vi "LV SciSDK DETACH BOARD.vi"(8 "error in (no error)":errorcluster, 9 "Board Handle In":T1) -> (0 "error out":errorcluster, 1 "SciSDK Handle":u64)   [LabVIEW 2021, in "SciSDK_Labview.lvlib"]
doc: "You need this VI to detach a board from SciSDK"
uses:
  SciSDK_Labview.lvlib
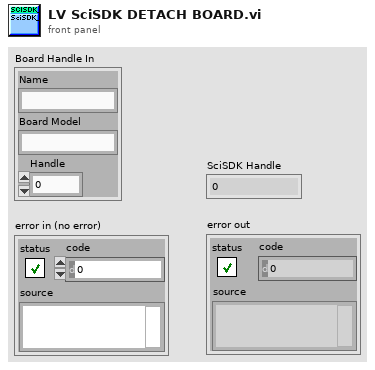
[diagram p1: front panel]
types:
  T1 = cluster{"Name":string, "Board Model":string, "Handle":u64}
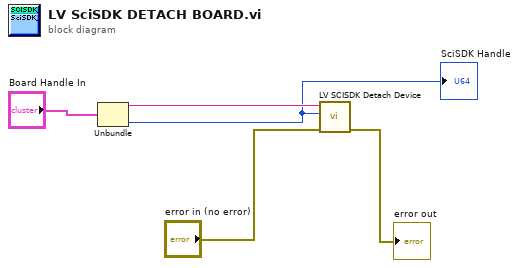
[diagram p0: block diagram]
diagram:
  n1 = Unbundle("Board Handle In") -> ("Name"=w4:string, "Handle"=w3:u64)  [unwired: 1 out]
  "SciSDK Handle" <- w3
  n2 = call "LV SCISDK Detach Device.vi"("error in (no error)"="error in (no error)", "handle"=w3, "name"=w4) -> ("error out"=→"error out":errorcluster)  [unwired: 7 in, 1 out]
